vi "List Input Reader.vi"(10 "file path (dialog if empty)":path=path "C:/git/AoC24/Day1/Tester.txt") -> (1 "all rows":string[](array[string]), 2 "Array":i32[][](array[numeric]))   [LabVIEW 2023]
uses:
  <vilib>/Utility/file.llb/Read Delimited Spreadsheet (string).vi
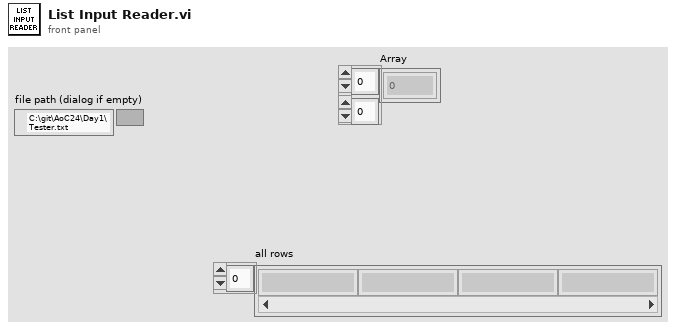
[diagram p1: front panel]
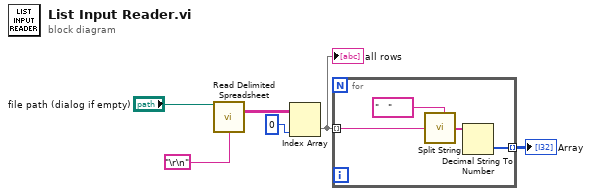
[diagram p0: block diagram]
diagram:
  n1 = call-poly <vilib>:"Read Delimited Spreadsheet.vi"("file path (dialog if empty)"="file path (dialog if empty)", "delimiter (\\t)"="\r\n") -> ("all rows"=w3:string[][])  [unwired: 8 in, 5 out]
  n2 = Index Array(array=w3, index (col)=0 ("disabled index (col)")) -> (element=w2:string[])  [unwired: 1 in]
  "all rows" <- w2
  n3 = for {
    tunnel: w2 -> [w10] mode=indexing
    tunnel: [w7] -> w1 mode=indexing
    n4 = call <vilib>:"Split String.vi"("Split Pattern"="   ", "Input String"=w10) -> ("Split String"=w8:string[])  [unwired: 5 in]
    n5 = Decimal String To Number(string=w8) -> (number=w7:i32[])  [unwired: 2 in, 1 out]
  }
  "Array" <- w1
